vi "Set Alarm 1 Hi.vi"(8 "error in":errorcluster, 10 "Alarm Hi":dbl, 11 "CnPt in":refnum<class "CnPt.lvclass">) -> (0 "error out":errorcluster, 3 "CnPt out":refnum<class "CnPt.lvclass">)   [LabVIEW 2015, in "CnPt.lvclass"]
uses:
  CnPt.lvclass
  <vilib>/MSR Consulting, LLC/General Reuse/Session APIs/Serial/Serial Session.lvclass
  CnPt.lvclass/CnPt.ctl
  <vilib>/MSR Consulting, LLC/General Reuse/Session APIs/Serial/Public/Asynchronous Write.vi
  <vilib>/MSR Consulting, LLC/General Reuse/Session APIs/Serial/Public/Asynchronous Read.vi
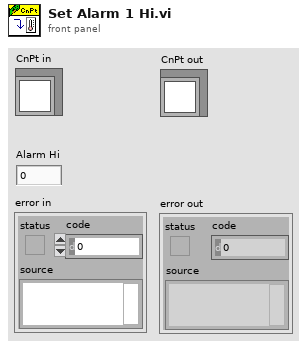
[diagram p1: front panel]
types:
  T1 = typedef "Serial Session.lvclass/Session Handle.ctl" = refnum<data-value>
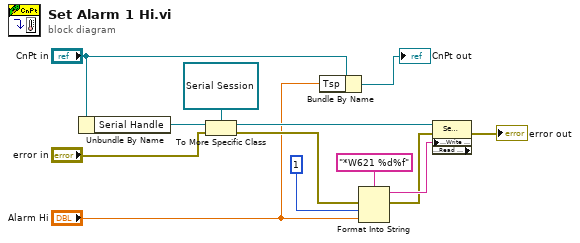
[diagram p0: block diagram]
diagram:
  n1 = Unbundle By Name("CnPt in") -> ("Serial Handle"=w13:T1)
  n2 = To More Specific Class(target class=refnum<data-value> refnum, reference=w13, error in="error in") -> (specific class reference=w11:refnum<data-value>, error out=w7:errorcluster)
  n3 = Bundle By Name(cluster="CnPt in", "Tsp"="Alarm Hi") -> (→"CnPt out":refnum<class "CnPt.lvclass">)
  n4 = Format Into String(format string="*W621 %d%f", error in=w7, 1, "Alarm Hi") -> (resulting string=w9:string, error out=w6:errorcluster)  [unwired: 1 in]
  n5 = property class="Serial Session" props=["Public:Write - Asynchronous", "Public:Read - Asynchronous"](reference=w11, error in=w6, "Public:Write - Asynchronous"=w9) -> (error out=→"error out":errorcluster)  [unwired: 2 out]
